vi "LAOnDone.vi"(8 "Error In":errorcluster, 11 "LiteAgent In":T1) -> (0 "Error Out":errorcluster, 3 "LiteAgent Out":T1)   [LabVIEW 2017, in "LiteAgentSDK.lvlib"]
uses:
  LiteAgentSDK.lvlib
  C:/Users/Jan/Projects/LiteAgentSDK-LabVIEW/Source/Bin/LiteAgentSDK.LabVIEW.dll
  Bin/LiteAgentSDK.LabVIEW.dll
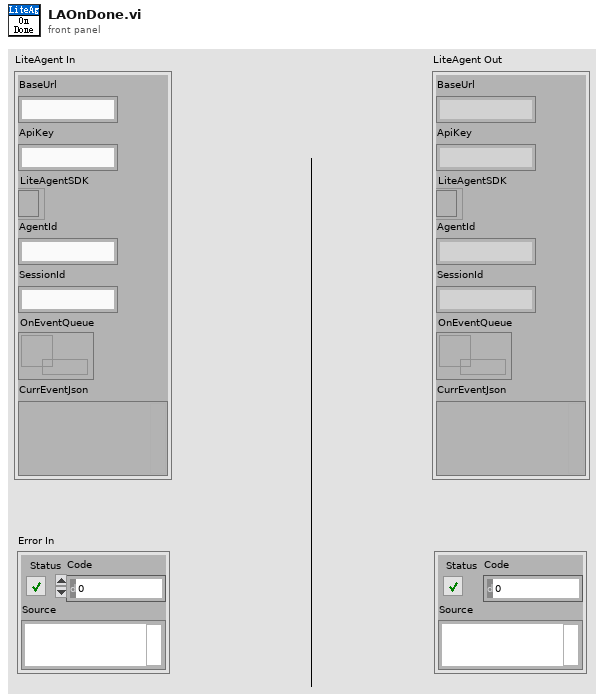
[diagram p1: front panel]
types:
  T1 = cluster{"BaseUrl":string, "ApiKey":string, "LiteAgentSDK":refnum<k24>, "AgentId":string, "SessionId":string, "OnEventQueue":refnum<queue>, "CurrEventJson":variant}
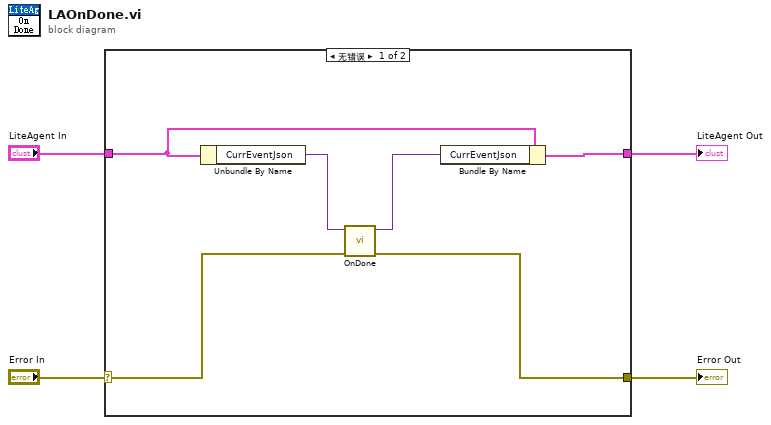
[diagram p0: block diagram]
diagram:
  n1 = case shown="无错误" "Error In" {
    selector: "Error In" -> [w7 w12]
    tunnel: [w6 w12] -> w3
    tunnel: "LiteAgent In" -> [w10 w11]
    tunnel: [w9 w11] -> w1
    frame No Error {
      n2 = Unbundle By Name(w10) -> ("CurrEventJson"=w8:variant)
      n3 = call "OnDone.vi"("Error In"=w7, "JSON Tree In"=w8) -> ("Error Out"=w6:errorcluster, "JSON Tree Out"=w5:variant)  [unwired: 8 in]
      n4 = Bundle By Name(cluster=w10, "CurrEventJson"=w5) -> (w9:T1)
    }
    frame Error {
    }
  }
  "Error Out" <- w3
  "LiteAgent Out" <- w1
